vi "Get Array of Move Button Configurations.vi"(8 "error in (no error)":errorcluster, 11 "VacuumLine Configuration in":refnum<class "VacuumLine Configuration.lvclass">) -> (0 "error out":errorcluster, 2 "Array of Move Button Configurations":T1[](array[typedef]) {"Target pos" format="%#_f mm"}, 3 "VacuumLine Configuration out":refnum<class "VacuumLine Configuration.lvclass">)   [LabVIEW 2016, in "Hardware.lvlib" / "VacuumLine.lvlib" / "VacuumLine Configuration.lvclass"]
uses:
  <userlib>/Common Components/Hardware/Abstract System/VacuumLine/VacuumLine Config/VacuumLine Configuration.lvclass
  <userlib>/Common Components/Hardware/Abstract System/VacuumLine/VacuumLine/Button Config Cluster.ctl
  <userlib>/Common Components/Hardware/Abstract System/VacuumLine/VacuumLine Config/VacuumLine Configuration.lvclass/VacuumLine Configuration.ctl
  <userlib>/Common Components/Hardware/Abstract System/VacuumLine/VacuumLine/VacuumLine.lvclass/VacuumLine.ctl
  <userlib>/Common Components/Hardware/Abstract System/VacuumLine/VacuumLine/VacuumLine.lvclass
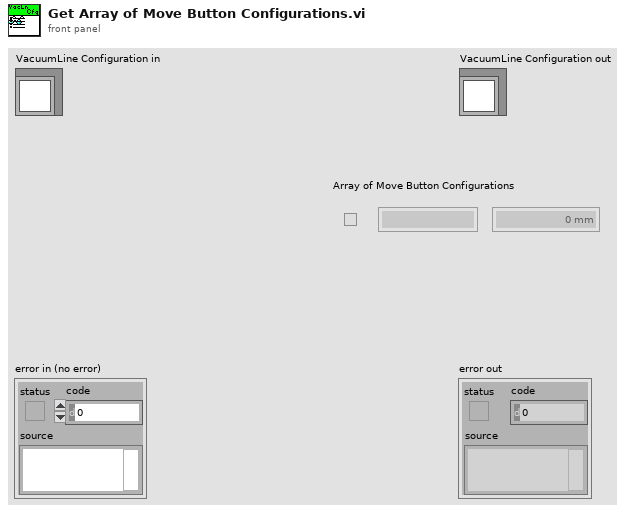
[diagram p1: front panel]
types:
  T1 = typedef "Hardware.lvlib/VacuumLine.lvlib/VacuumLine.lvclass/Button Config Cluster.ctl" = cluster{"Enabled?":bool, "Text on button":string, "Target pos":dbl}
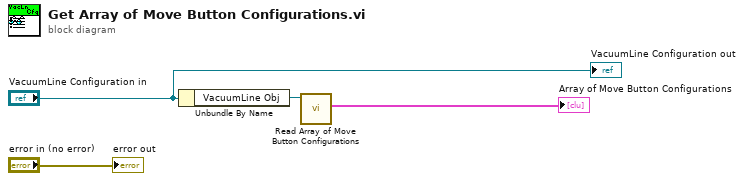
[diagram p0: block diagram]
diagram:
  n1 = Unbundle By Name("VacuumLine Configuration in") -> ("VacuumLine Obj"=w3:refnum<class "VacuumLine.lvclass">)
  n2 = call <userlib>:"Read Array of Move Button Configurations.vi"("VacuumLine in"=w3) -> ("Array of Move Button Configurations"=→"Array of Move Button Configurations":T1[])  [unwired: 9 in, 1 out]
  "error out" <- "error in (no error)"
  "VacuumLine Configuration out" <- "VacuumLine Configuration in"
